vi "Custom_Append VI Icon to Report (refnum).vi"(0 "report in":refnum<class "NI_report.lvclass">, 2 "image format (jpeg)":enum32{"PNG", "JPEG", "GIF"}(ring)=enum."JPEG", 5 "VI":refnum<vi>, 7 "alignment (default)":T1, 9 "caption or alternative string":string, 11 "error in (no error)":errorcluster, 12 "MS Office parameters":T2) -> (4 "report out":refnum<class "NI_report.lvclass">, 6 "VI out":refnum<vi>, 8 "start out (Word)":i32, 10 "end out (Word)":i32, 15 "error out":errorcluster)   [LabVIEW 2019]
doc: "Appends the icon of the VI you specify in <B>VI</B> to a report. Wire data to the <B>VI</B> input to determine the polymorphic instance to use or manually select the instance."
uses:
  <vilib>/Utility/NIReport.llb/NI_report.lvclass
  <vilib>/Utility/NIReport.llb/HTML Report Image Alignment.ctl
  <vilib>/Utility/NIReport.llb/NI_ReportGenerationCore.lvlib
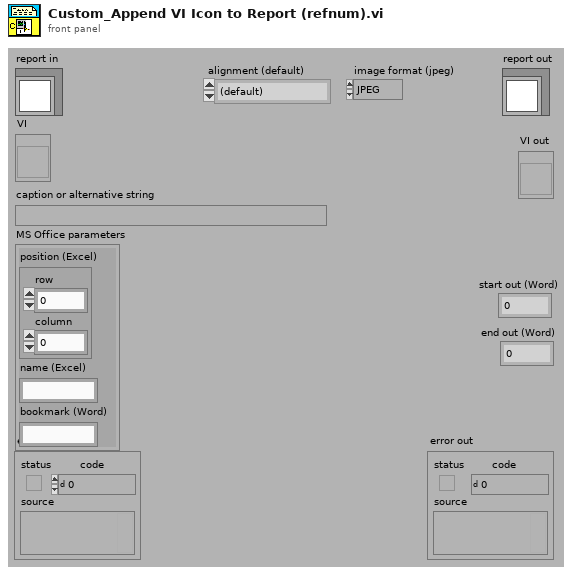
[diagram p1: front panel]
types:
  T1 = typedef "NI_ReportGenerationCore.lvlib/HTML Report Image Alignment.ctl" = enum16{"(default)", "LEFT", "RIGHT", "TOP", "TEXTTOP", "MIDDLE", "ABSMIDDLE", "BASELINE", "BOTTOM", "ABSBOTTOM"}
  T2 = cluster{"position (Excel)":cluster{"row":i32, "column":i32}, "name (Excel)":string, "bookmark (Word)":string}
  T3 = enum32{"invalid app kind", "Development System", "Run Time System", "Student Edition", "Embedded LabVIEW", "Evaluation", "Custom"}
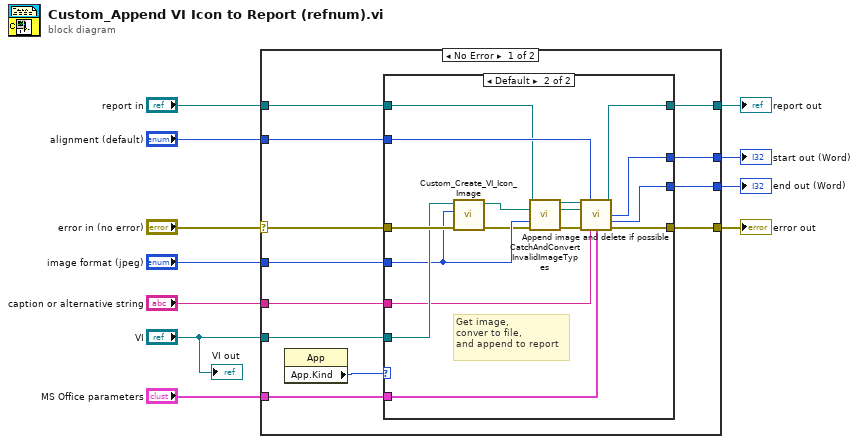
[diagram p0: block diagram]
diagram:
  n1 = case shown="No Error" "error in (no error)" {
    selector: "error in (no error)" -> [w23 w43]
    tunnel: [w21 w43] -> w10
    tunnel: "report in" -> [w14 w42]
    tunnel: "VI" -> [w22 _]
    tunnel: "image format (jpeg)" -> [w20 _]
    tunnel: "MS Office parameters" -> [w19 _]
    tunnel: "alignment (default)" -> [w18 _]
    tunnel: "caption or alternative string" -> [w17 _]
    tunnel: [w16 _] -> w3
    tunnel: [w15 _] -> w2
    tunnel: [w13 w42] -> w1
    frame No Error {
      n2 = property class="App"() -> ("App.Kind"=w12:T3)  [unwired: 2 in, 2 out]
      n3 = case shown="Default" w12 {
        tunnel: w23 -> [w24 w41]
        tunnel: w22 -> [_ w40]
        tunnel: [w24 w39] -> w21
        tunnel: w20 -> [_ w35]
        tunnel: w19 -> [_ w33]
        tunnel: w18 -> [_ w32]
        tunnel: w17 -> [_ w31]
        tunnel: [_ w30] -> w16
        tunnel: [_ w29] -> w15
        tunnel: w14 -> [w25 w27]
        tunnel: [w25 w26] -> w13
        frame "Run Time System" {
        }
        frame Default {
          # "Get image,\nconver to file,\nand append to report"
          n4 = call "Custom_Create_VI_Icon_Image.vi"("error in (no error)"=w41, "Image Format (jpeg)"=w35, "VI"=w40) -> ("error out"=w34:errorcluster, "Path to image"=w28:path)  [unwired: 7 in]
          n5 = call-dynamic "CatchAndConvertInvalidImageTypes.vi"("report in"=w27, "path to image"=w28, "image format (jpeg)"=w35, "error in (no error)"=w34) -> ("report out"=w36:refnum<class "NI_report.lvclass">, "path to image out"=w37:path, "error out"=w38:errorcluster)  [unwired: 9 in]
          n6 = call-dynamic "Append image and delete if possible.vi"("report in"=w36, "alignment (default)"=w32, "path to image"=w37, "error in (no error)"=w38, "caption or alternative string"=w31, "MS Office parameters"=w33) -> ("report out"=w26:refnum<class "NI_report.lvclass">, "start out Word)"=w30:i32, "end out Word)"=w29:i32, "error out"=w39:errorcluster)  [unwired: 6 in]
        }
      }
    }
    frame Error {
    }
  }
  "error out" <- w10
  "report out" <- w1
  "start out (Word)" <- w3
  "end out (Word)" <- w2
  "VI out" <- "VI"
